vi "Get Supported Targets.vi"(8 "error in":errorcluster, 11 "RTResourceUtilitzation configuration in":refnum<class "RTResourceUtilitzation configuration.lvclass">) -> (0 "error out":errorcluster, 2 "supported targets":T1[](array[typedef]), 3 "RTResourceUtilitzation configuration out":refnum<class "RTResourceUtilitzation configuration.lvclass">)   [LabVIEW 2014, in "RTResourceUtilitzation configuration.lvclass"]
doc: "Provides an interface for determining the targets supported by a given module configuration/runtime class pairing. This should be overridden by any useful child class."
uses:
  RTResourceUtilitzation configuration.lvclass
  <vilib>/NI/Tag Bus Module Framework/root configuration/Target Types.ctl
  <vilib>/NI/Tag Bus Module Framework/root configuration/TBM configuration.lvclass
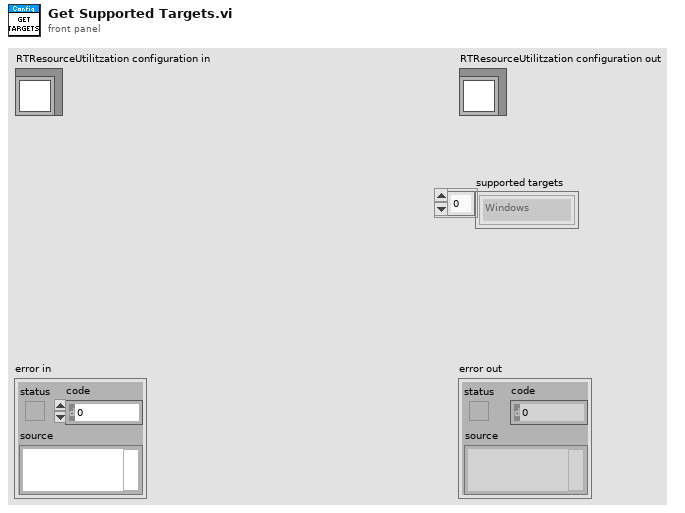
[diagram p1: front panel]
types:
  T1 = typedef "TBM configuration.lvclass/Target Types.ctl" = enum16{"Windows", "Mac", "Linux", "Linux RT ARM", "VxWorks", "Pharlap", "Other", "Linux RT x64"}
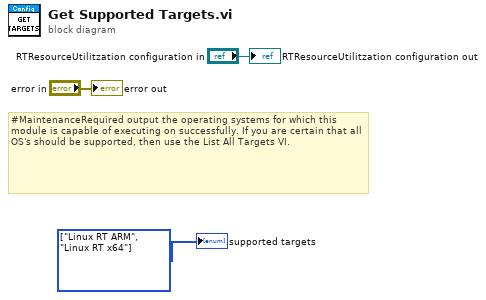
[diagram p0: block diagram]
diagram:
  w1 = T1[] [enum."Linux RT ARM", enum."Linux RT x64"] items=["Windows", "Mac", "Linux", "Linux RT ARM", "VxWorks", "Pharlap", "Other", "Linux RT x64"] ("supported targets")
  # "#MaintenanceRequired output the operating systems for which this module is capable of executing on successfully. If you are certain that all OS's should be supported, then use the List All Targets VI."
  "error out" <- "error in"
  "RTResourceUtilitzation configuration out" <- "RTResourceUtilitzation configuration in"
  "supported targets" <- w1
